vi "Get WAMP Message Type.vi"(10 "error in (no error)":errorcluster, 11 "JSON":string) -> (0 "<JSON>":string[](array[string]) caption="<JSON>Elements", 1 "Message Codes":T2=1 items=["HELLO"=1, "WELCOME"=2, "ABORT"=3, "GOODBYE"=6, "ERROR"=8, "PUBLISH"=16, "PUBLISHED"=17, "SUBSCRIBE"=32, "SUBSCRIBED"=33, "UNSUBSCRIBE"=34, "UNSUBSCRIBED"=35, "EVENT"=36, "CALL"=48, "RESULT"=59, "REGISTER"=64, "REGISTERED"=65, "UNREGISTER"=66, "UNREGISTERED"=67, "INVOCATION"=68, "YIELD"=70], 2 "error out":errorcluster, 3 "WAMP Message":T1 {"Message Codes" items=["HELLO"=1, "WELCOME"=2, "ABORT"=3, "GOODBYE"=6, "ERROR"=8, "PUBLISH"=16, "PUBLISHED"=17, "SUBSCRIBE"=32, "SUBSCRIBED"=33, "UNSUBSCRIBE"=34, "UNSUBSCRIBED"=35, "EVENT"=36, "CALL"=48, "RESULT"=59, "REGISTER"=64, "REGISTERED"=65, "UNREGISTER"=66, "UNREGISTERED"=67, "INVOCATION"=68, "YIELD"=70]})   [LabVIEW 2020, in "wamplv.lvlib" / "WAMP Client.lvclass"]
uses:
  WAMP Client.lvclass
  TypeDef/WAMP Message Codes.ctl
  TypeDef/WAMP Received Message.ctl
  WAMP Client.lvclass/WAMP Client.ctl
  <vilib>/JDP Science/JSONtext/JSONtext.lvlib
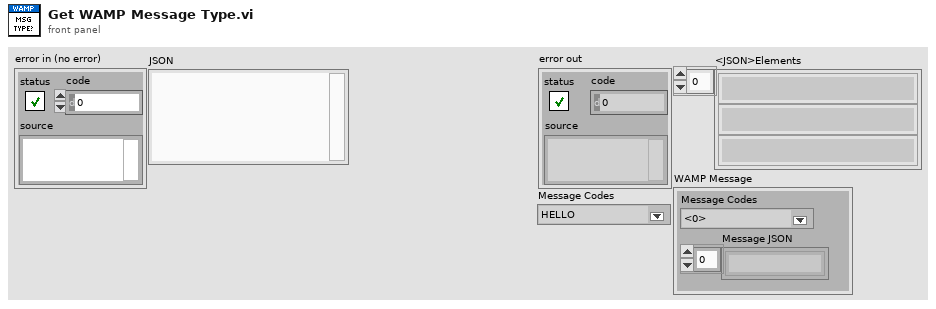
[diagram p1: front panel]
types:
  T1 = typedef "wamplv.lvlib/WAMP Client.lvclass/WAMP Received Message.ctl" = cluster{"Message JSON":string[], "Message Codes":T2}
  T2 = typedef "wamplv.lvlib/WAMP Client.lvclass/WAMP Message Codes.ctl" = u16
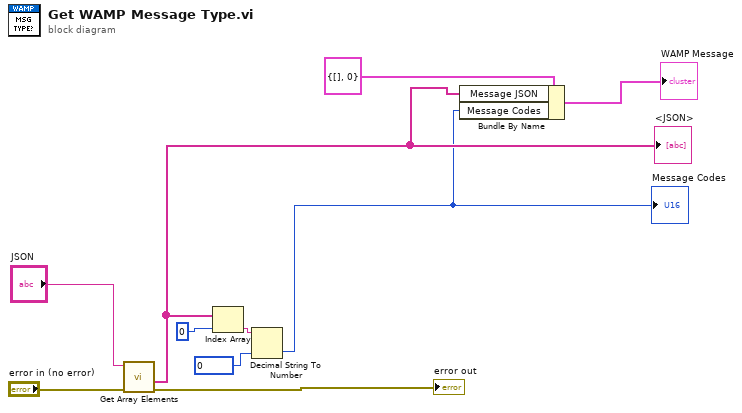
[diagram p0: block diagram]
diagram:
  w5 = T2 0 items=["HELLO"=1, "WELCOME"=2, "ABORT"=3, "GOODBYE"=6, "ERROR"=8, "PUBLISH"=16, "PUBLISHED"=17, "SUBSCRIBE"=32, "SUBSCRIBED"=33, "UNSUBSCRIBE"=34, "UNSUBSCRIBED"=35, "EVENT"=36, "CALL"=48, "RESULT"=59, "REGISTER"=64, "REGISTERED"=65, "UNREGISTER"=66, "UNREGISTERED"=67, "INVOCATION"=68, "YIELD"=70] ("Message Codes")
  n1 = call <vilib>:"Get Array Elements.vi"("error in (no error)"="error in (no error)", "JSON"="JSON") -> ("error out"=→"error out":errorcluster, "<JSON>"=w3:string[])  [unwired: 7 in, 1 out]
  "<JSON>" <- w3
  n2 = Index Array(array=w3, index=0) -> (element=w7:string)
  n3 = Decimal String To Number(string=w7, default (0L)=w5) -> (number=w2:u16)  [unwired: 1 in, 1 out]
  "Message Codes" <- w2
  n4 = Bundle By Name(cluster=T1 {"Message JSON"=[], "Message Codes"=0} ("Cluster"), "Message JSON"=w3, "Message Codes"=w2) -> (→"WAMP Message":T1)
